vi "UpdateCameraInfoWithUserCfg.vi"(7 "found":bool, 10 "channel":T1, 11 "camera info":T4) -> (3 "camera info":T4)   [LabVIEW 2017, in "IrManageCameras.lvlib"]
uses:
  <vilib>/addons/InsightCM/Devices/Shared/Ir/IrManageCameras/IrManageCameras.lvlib
  <vilib>/addons/InsightCM/Devices/Shared/Ir/IrManageCameras/controls/camera.ctl
  <vilib>/addons/InsightCM/MessageBus/Base/controls/R2_Channel.ctl
  <vilib>/addons/InsightCM/MessageBus/Base/controls/KeyValuePair.ctl
  <vilib>/addons/InsightCM/MessageBus/Base/controls/Metric.ctl
  <vilib>/addons/InsightCM/Utilities/PropertyHelpers/PropertyHelpers.lvlib
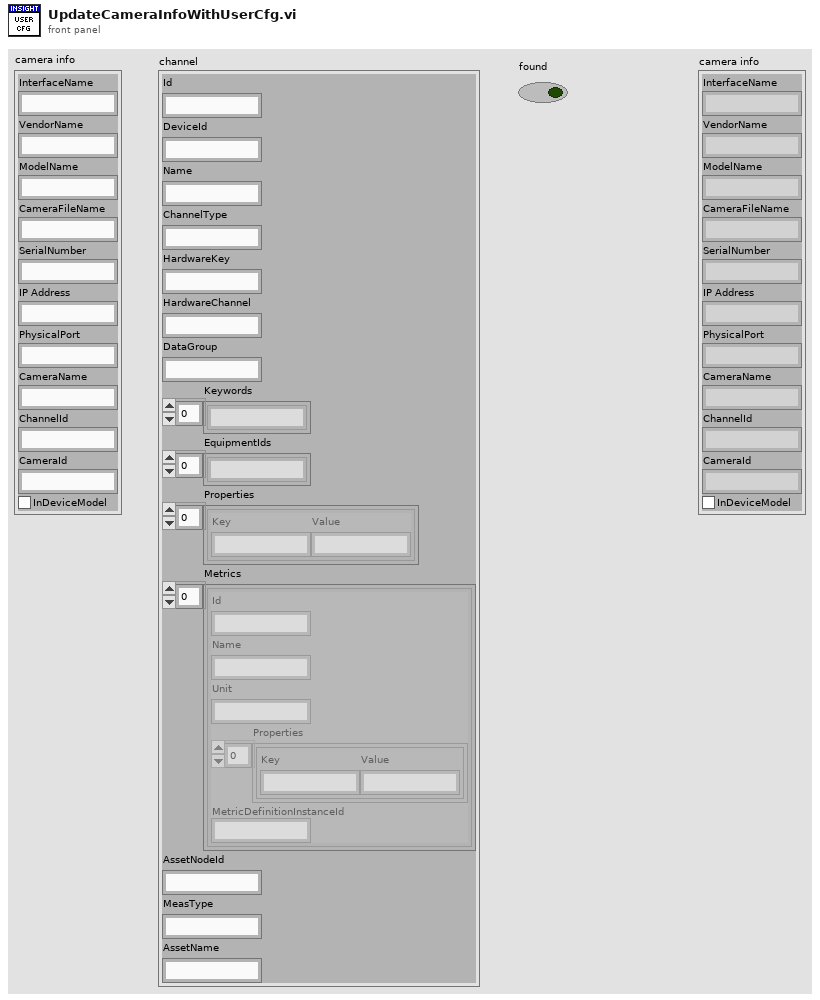
[diagram p1: front panel]
types:
  T1 = typedef "R2_Channel.ctl" = cluster{"Id":string, "DeviceId":string, "Name":string, "ChannelType":string, "HardwareKey":string, "HardwareChannel":string, "DataGroup":string, "Keywords":string[], "EquipmentIds":string[], "Properties":T2[], "Metrics":T3[], "AssetNodeId":string, "MeasType":string, "AssetName":string}
  T2 = typedef "KeyValuePair.ctl" = cluster{"Key":string, "Value":string}
  T3 = typedef "Metric.ctl" = cluster{"Id":string, "Name":string, "Unit":string, "Properties":T2[], "MetricDefinitionInstanceId":string}
  T4 = typedef "IrManageCameras.lvlib/camera.ctl" = cluster{"InterfaceName":string, "VendorName":string, "ModelName":string, "CameraFileName":string, "SerialNumber":string, "IP Address":string, "PhysicalPort":string, "CameraName":string, "ChannelId":string, "CameraId":string, "InDeviceModel":bool}
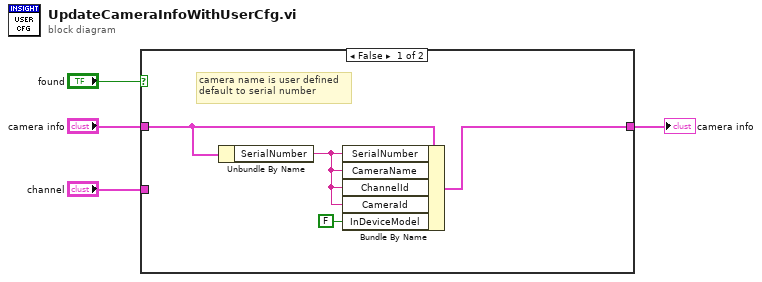
[diagram p0: block diagram]
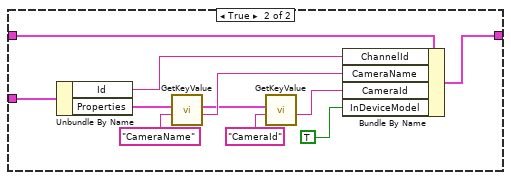
[diagram p2: hidden frame]
diagram:
  n1 = case shown="False" "found" {
    tunnel: "camera info" -> [w8 w18]
    tunnel: "channel" -> [_ w19]
    tunnel: [w7 w17] -> w2
    frame False {
      # "camera name is user defined\ndefault to serial number"
      n2 = Unbundle By Name(w8) -> ("SerialNumber"=w6:string)
      n3 = Bundle By Name(cluster=w8, "SerialNumber"=w6, "CameraName"=w6, "ChannelId"=w6, "CameraId"=w6, "InDeviceModel"=FALSE) -> (w7:T4)
    }
    frame True {
      n4 = Unbundle By Name(w19) -> ("Id"=w16:string, "Properties"=w15:T2[])
      n5 = call <vilib>:"GetKeyValue.vi"("key"="CameraName", "key value pairs"=w15) -> ("value"=w14:string, "key value pairs out"=w11:T2[])  [unwired: 7 in, 1 out]
      n6 = call <vilib>:"GetKeyValue.vi"("key"="CameraId", "key value pairs"=w11) -> ("value"=w10:string)  [unwired: 7 in, 2 out]
      n7 = Bundle By Name(cluster=w18, "ChannelId"=w16, "CameraName"=w14, "CameraId"=w10, "InDeviceModel"=TRUE) -> (w17:T4)
    }
  }
  "camera info" <- w2
